vi "Teleop.vi"(10 "Match Info":T1={"Autonomous Elapsed Seconds"=0.0, "TeleOp Elapsed Seconds"=0.0, "Disabled Elapsed Seconds"=0.0, "Visited Autonomous"=FALSE, "Visited TeleOp"=FALSE, "Visited Disabled"=FALSE, "Autonomous Settings"={"Autonomous Style"=enum."Independent", "VI Refnum"=refnum}}, 11 "Call Context":T2) -> ()   [LabVIEW 2017]
doc: "This VI is called for each TeleOp packet received from the DS where the robot is not disabled. It is often used to read from the joysticks and update I/O or to update setpoints for timed control loops. It should complete and return within 20 milliseconds or it may miss DS packets."
uses:
  <vilib>/Rock Robotics/WPI/DriverStation/WPI_DriverStationDerivedRobotMode.ctl
  <vilib>/Rock Robotics/WPI/DriverStation/WPI_DriverStationMatch Info.ctl
  <vilib>/Rock Robotics/WPI/Solenoid/WPI_SolenoidValue.ctl
  Robot Global Data.vi
  <vilib>/Rock Robotics/Network Tables/NT Write Boolean Array.vi
  <vilib>/Rock Robotics/Network Tables/NT Write Numeric Array.vi
  <vilib>/Rock Robotics/WPI/Utilities/WPI_GetSetVariantRefNum.vi
  <vilib>/Rock Robotics/Network Tables/NT Read Boolean.vi
  <vilib>/Rock Robotics/Network Tables/NT Read String.vi
  <vilib>/Rock Robotics/WPI/Solenoid/WPI_SolenoidSetEnum.vi
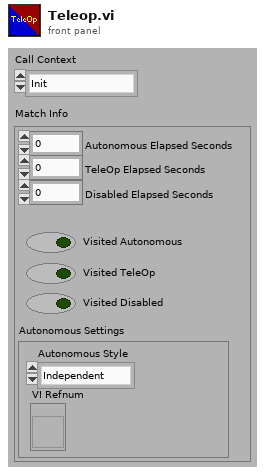
[diagram p1: front panel]
types:
  T1 = typedef "WPI_DriverStationMatch Info.ctl" = cluster{"Autonomous Elapsed Seconds":dbl, "TeleOp Elapsed Seconds":dbl, "Disabled Elapsed Seconds":dbl, "Visited Autonomous":bool, "Visited TeleOp":bool, "Visited Disabled":bool, "Autonomous Settings":cluster{"Autonomous Style":enum16{"Iterative", "Independent"}, "VI Refnum":refnum<vi>}}
  T2 = typedef "WPI_DriverStationDerivedRobotMode.ctl" = enum16{"Init", "Execute", "Stop"}
  T3 = enum16{"1 Xbox Controller", "2 Xbox Controllers"}
  T4 = typedef "TeleopCommands.ctl" = cluster{"Drive Axes":dbl[], "Shooter Forwards":bool, "Shooter Reverse":bool, "Intake Forwards":bool, "Intake Reverse":bool, "Lift Forwards":bool, "Lift Reverse":bool, "Agitator Forwards":bool, "Agitator Reverse":bool, "Left Gear Angle":bool, "Mid Gear Angle":bool, "Right Gear Angle":bool, "Shooter Distance":bool, "Vision Align":bool, "Place Gear":bool, "Command Stop":bool, "Reset Gyro":bool, "Jog Mode?":bool, "Lift Override":bool, "Lift Power":dbl}
  T5 = typedef "WPI_JoystickDevRef.ctl" = cluster{"Device":T6}
  T6 = typedef "WPI_JoystickDeviceEnum.ctl" = enum16{"USB 0", "USB 1", "USB 2", "USB 3", "USB 4", "USB 5"}
  T7 = cluster{"Yaw":dbl, "Roll":dbl, "Pitch":dbl, "Heading":dbl, "Fused Heading":dbl}
  T8 = typedef "WPI_MotorControlDeviceRef.ctl" = cluster{"DeviceStatus":errorcluster, "Type":T9, "PWM":cluster{"PWM Channel":T10, "DeadBand":T11}, "CAN":cluster{"Device Number":u8, "SetOutput VI Ref":variant, "GetOutput VI Ref":variant, "Enable VI Ref":variant, "Disable VI Ref":variant, "Data":variant}, "Invert":bool, "DIO PWM":cluster{"PWM \"Enable\" Channel":T10, "DIOChannel":T12, "PWM Rate":dbl}}
  T9 = typedef "WPI_MotorControlType.ctl" = enum16{"PWM", "CAN", "DIO PWM"}
  T10 = typedef "FPGA_DIOPWMChannel.ctl" = enum8{"PWM 0", "PWM 1", "PWM 2", "PWM 3", "PWM 4", "PWM 5", "PWM 6", "PWM 7", "PWM 8", "PWM 9", "PWM MXP 0", "PWM MXP 1", "PWM MXP 2", "PWM MXP 3", "PWM MXP 4", "PWM MXP 5", "PWM MXP 6", "PWM MXP 7", "PWM MXP 8", "PWM MXP 9", "Invalid"}
  T11 = typedef "WPI_PWMDeadband.ctl" = cluster{"Name":string, "maxPositivePwm":i32, "minPositivePwm":i32, "centerPwm":i32, "maxNegativePwm":i32, "minNegativePwm":i32, "angularRange":u16}
  T12 = typedef "FPGA_DIOChannel.ctl" = enum8{"DIO 0", "DIO 1", "DIO 2", "DIO 3", "DIO 4", "DIO 5", "DIO 6", "DIO 7", "DIO 8", "DIO 9", "DIO MXP 0", "DIO MXP 1", "DIO MXP 2", "DIO MXP 3", "DIO MXP 4", "DIO MXP 5", "DIO MXP 6", "DIO MXP 7", "DIO MXP 8", "DIO MXP 9", "DIO MXP 10", "DIO MXP 11", "DIO MXP 12", "DIO MXP 13", "DIO MXP 14", "DIO MXP 15", "SPI Port CS1", "SPI Port CS2", "SPI Port CS3", "SPI Port MISO", "SPI Port MOSI", "Invalid"}
  T13 = typedef "WPI_SolenoidDevRef.ctl" = cluster{"DevStatus":errorcluster, "Pneumatics Control Module":u8, "Forward Solenoid Channel":T14, "Reverse Solenoid Channel":T14}
  T14 = typedef "WPI_SolenoidChannel.ctl" = enum8{"Solenoid 0", "Solenoid 1", "Solenoid 2", "Solenoid 3", "Solenoid 4", "Solenoid 5", "Solenoid 6", "Solenoid 7", "Invalid"}
  T15 = typedef "WPI_SolenoidValue.ctl" = enum16{"Off", "On", "Forward", "Reverse"}
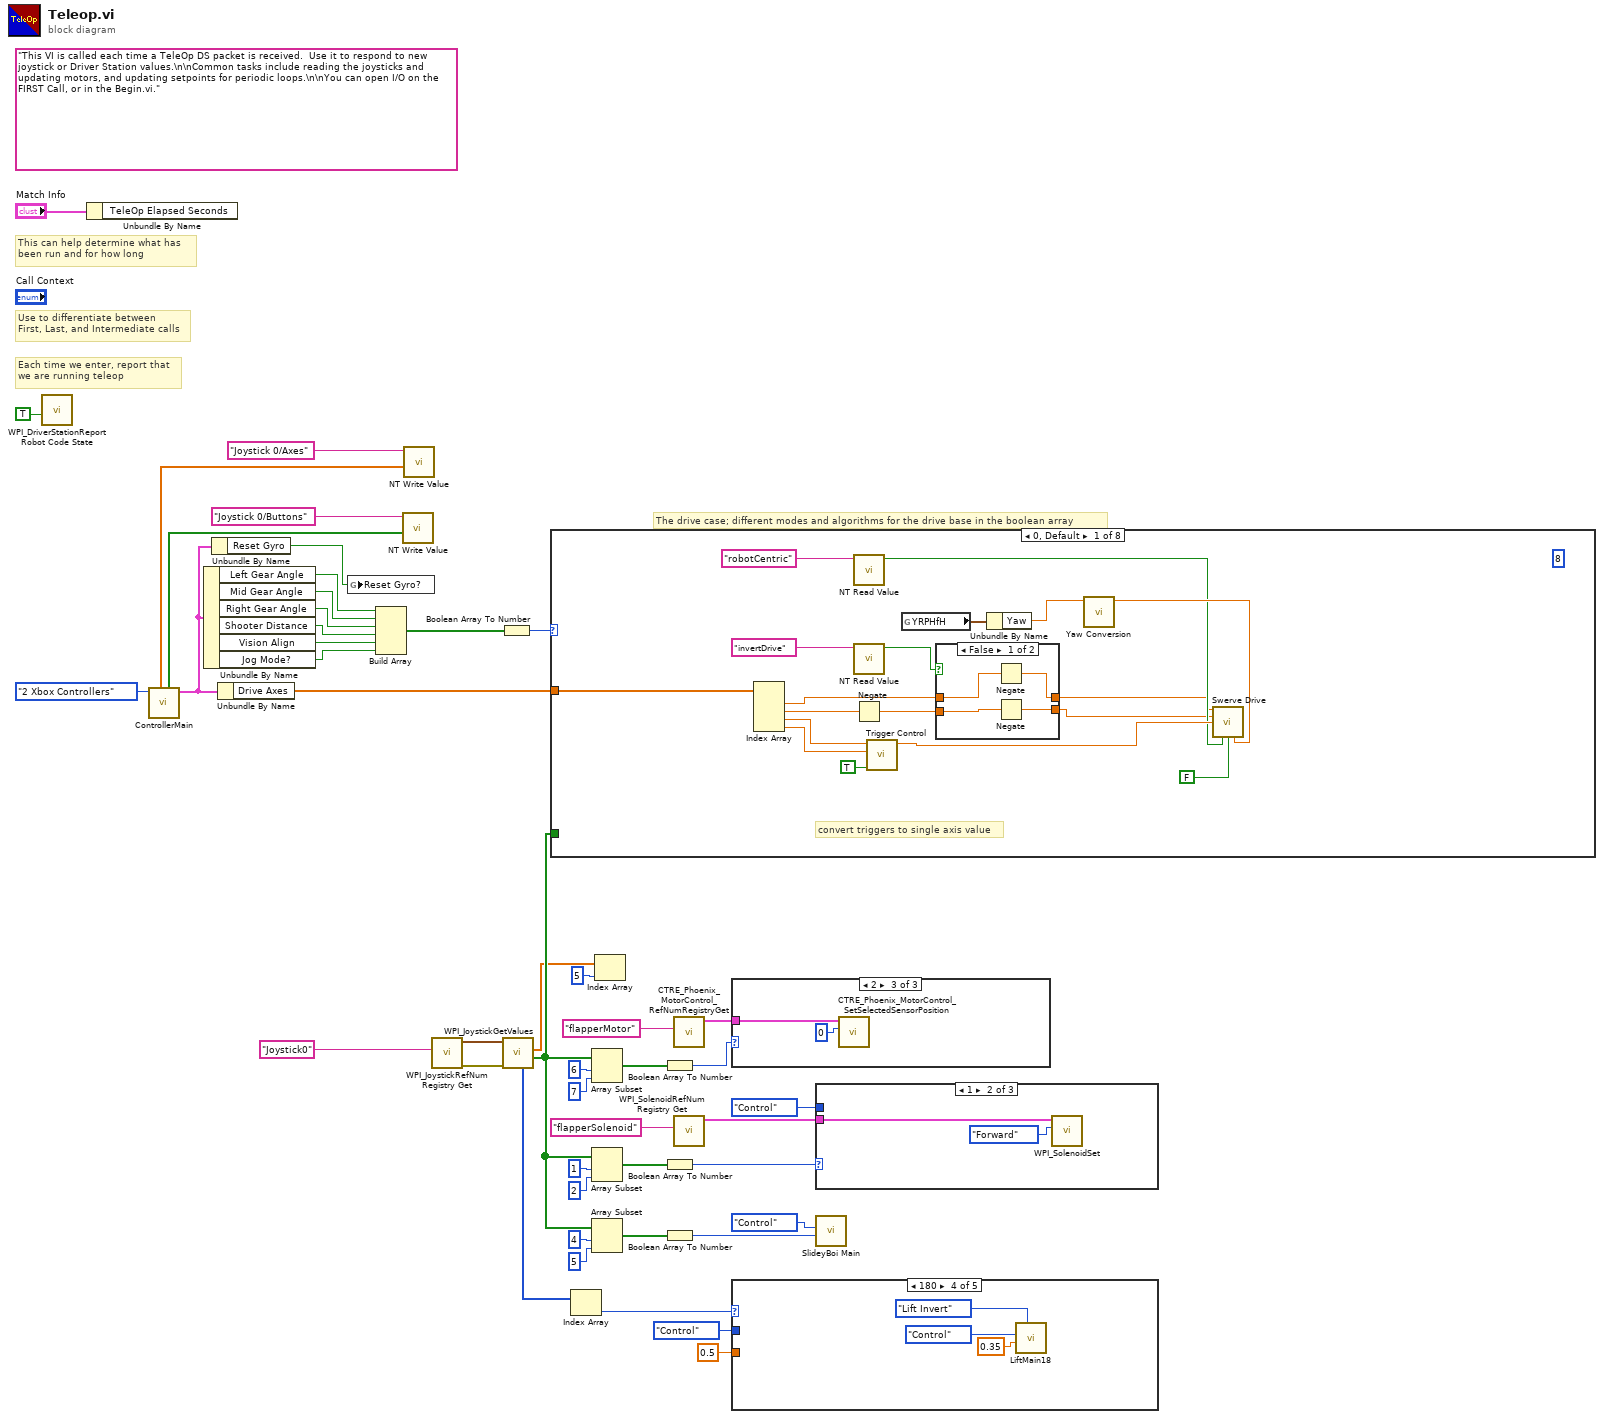
[diagram p0: block diagram]
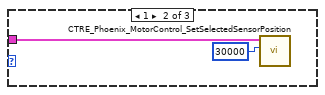
[diagram p3: hidden frame]
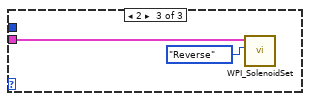
[diagram p5: hidden frame]
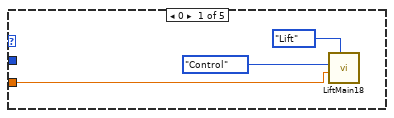
[diagram p6: hidden frame]
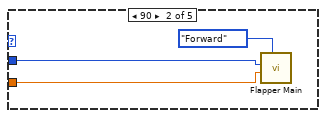
[diagram p7: hidden frame]
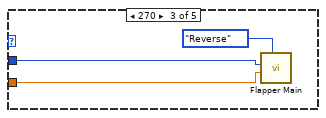
[diagram p8: hidden frame]
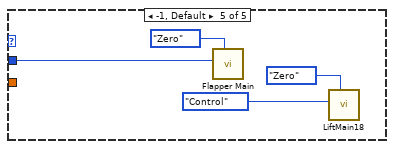
[diagram p9: hidden frame]
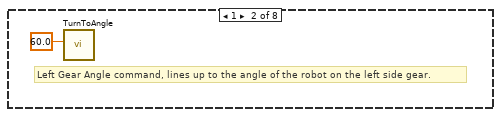
[diagram p11: hidden frame]
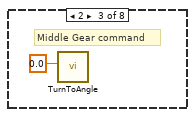
[diagram p12: hidden frame]
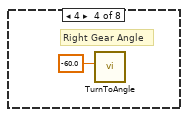
[diagram p13: hidden frame]
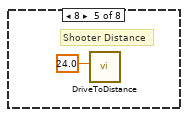
[diagram p14: hidden frame]
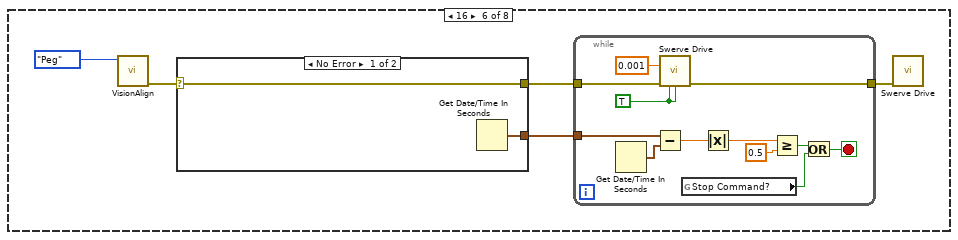
[diagram p15: hidden frame]
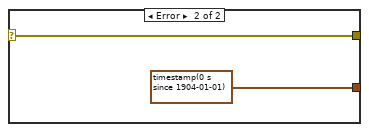
[diagram p16: hidden frame]
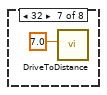
[diagram p17: hidden frame]
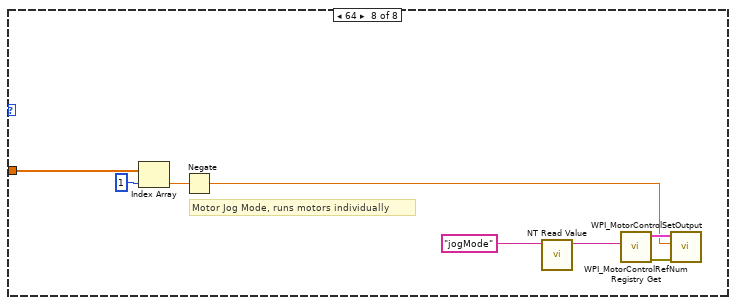
[diagram p18: hidden frame]
diagram:
  (unwired) "This VI is called each time a TeleOp DS packet is received.  Use it to respond to new joystick or Driver Station values.\n\nCommon tasks include reading the joysticks and updating motors, and updating setpoints for periodic loops.\n\nYou can open I/O on the FIRST Call, or in the Begin.vi."
  # "The drive case; different modes and algorithms for the drive base in the boolean array"
  # "Each time we enter, report that\nwe are running teleop"
  # "Use to differentiate between\nFirst, Last, and Intermediate calls"
  # "This can help determine what has\nbeen run and for how long"
  n1 = call <vilib>:"WPI_DriverStationReport Robot Code State.vi"("TeleOp"=TRUE ("Autonomous")) -> ()  [unwired: 10 in, 1 out]
  n2 = Unbundle By Name("Match Info") -> ()  [unwired: 1 out]
  n3 = call "ControllerMain.vi"("Control Mode"=T3."2 Xbox Controllers") -> ("Robot Inputs"=w39:T4, "Stick0 Buttons"=w42:bool[], "Stick0 Axes"=w43:dbl[])  [unwired: 5 in, 3 out]
  n4 = Unbundle By Name(w39) -> ("Left Gear Angle"=w37:bool, "Mid Gear Angle"=w36:bool, "Right Gear Angle"=w35:bool, "Shooter Distance"=w34:bool, "Vision Align"=w33:bool, "Jog Mode?"=w32:bool)
  n5 = Unbundle By Name(w39) -> ("Reset Gyro"=w38:bool)
  n6 = Unbundle By Name(w39) -> ("Drive Axes"=w29:dbl[])
  n7 = global write "Robot Global Data.vi" "Reset Gyro?"(w38) -> ()
  n8 = Build Array(w37, w36, w35, w34, w33, w32) -> (w31:bool[])
  n9 = call-poly <vilib>:"NT Write Value.vi"("Boolean Array"=w42, "Name"="Joystick 0/Buttons") -> ()  [unwired: 9 in, 1 out]
  n10 = call-poly <vilib>:"NT Write Value.vi"("Numeric Array"=w43, "Name"="Joystick 0/Axes") -> ()  [unwired: 9 in, 1 out]
  n11 = call <vilib>:"WPI_JoystickRefNum Registry Get.vi"("refnum name"="Joystick0") -> ("error out"=w27:errorcluster, "JoystickDevRef"=w26:T5)  [unwired: 9 in]
  n12 = Boolean Array To Number(Boolean array=w31) -> (number=w30:u32)
  n13 = call <vilib>:"WPI_JoystickGetValues.vi"("error in (no error)"=w27, "JoystickDevRef"=w26) -> ("Buttons"=w4:bool[], "Axes"=w3:dbl[], "POVs"=w25:i16[])  [unwired: 5 in, 2 out]
  n14 = case shown="0, Default" w30 {
    tunnel: w29 -> [w62 _ _ _ _ _ _ w104]
    tunnel: w4 -> [_ _ _ _ _ _ _ _]
    frame 0, Default {
      (unwired) 8 ("index")
      # "convert triggers to single axis value"
      n15 = Index Array(array=w62) -> (element #1=w54:dbl, element #2=w52:dbl, element #3=w61:dbl, element #4=w60:dbl)  [unwired: 4 in]
      n16 = call-poly <vilib>:"NT Read Value.vi"("Name"="robotCentric") -> ("Boolean"=w49:bool)  [unwired: 9 in, 1 out]
      n17 = call-poly <vilib>:"NT Read Value.vi"("Name"="invertDrive") -> ("Boolean"=w63:bool)  [unwired: 9 in, 1 out]
      n18 = Negate(x=w52) -> (-x=w53:dbl)
      n19 = call "Trigger Control.vi"("Invert?"=TRUE, "Axis 2 In"=w60, "Axis 1 In"=w61) -> ("Axis Out"=w56:dbl)  [unwired: 8 in]
      n20 = global read "Robot Global Data.vi" "YRPHfH"() -> (w58:T7)
      n21 = case shown="False" w63 {
        tunnel: w53 -> [w68 w70]
        tunnel: w54 -> [w67 w69]
        tunnel: [w66 w70] -> w48
        tunnel: [w65 w69] -> w47
        frame False {
          n22 = Negate(x=w67) -> (-x=w65:dbl)
          n23 = Negate(x=w68) -> (-x=w66:dbl)
        }
        frame True {
        }
      }
      n24 = Unbundle By Name(w58) -> ("Yaw"=w51:dbl)
      n25 = call "Yaw Conversion.vi"("Input"=w51) -> ("Output"=w50:dbl)  [unwired: 10 in]
      n26 = call "Swerve Drive.vi"("X"=w47, "Y"=w48, "Z"=w56, "Robot Centric?"=w49, "Autonomous?"=FALSE ("Robot Centric?"), "Yaw"=w50) -> ()  [unwired: 5 in, 5 out]
    }
    frame 1 {
      # "Left Gear Angle command, lines up to the angle of the robot on the left side gear."
      n27 = call "TurnToAngle.vi"("Target Angle"=60.0) -> ()  [unwired: 10 in, 1 out]
    }
    frame 2 {
      # "Middle Gear command"
      n28 = call "TurnToAngle.vi"("Target Angle"=0.0) -> ()  [unwired: 10 in, 1 out]
    }
    frame 4 {
      # "Right Gear Angle"
      n29 = call "TurnToAngle.vi"("Target Angle"=-60.0) -> ()  [unwired: 10 in, 1 out]
    }
    frame 8 {
      # "Shooter Distance"
      n30 = call "DriveToDistance.vi"("Setpoint"=24.0) -> ()  [unwired: 10 in, 1 out]
    }
    frame 16 {
      n31 = call "VisionAlign.vi"("Control Mode"=enum16{"Boiler", "Peg"}."Peg") -> ("Error Out"=w78:errorcluster)  [unwired: 10 in]
      n32 = case shown="No Error" w78 {
        selector: w78 -> [w93 w94]
        tunnel: [w93 w94] -> w76
        tunnel: [w92 timestamp(0 s since 1904-01-01)] -> w77
        frame No Error {
          n33 = Get Date/Time In Seconds() -> (seconds since 1Jan1904=w92:timestamp)
        }
        frame Error {
        }
      }
      n34 = while {
        tunnel: w77 -> [w91]
        tunnel: w76 -> [w85]
        tunnel: [w80] -> w75
        stop <- w81 stop-if-true
        w86 = TRUE ("Robot Centric?")
        n35 = Get Date/Time In Seconds() -> (seconds since 1Jan1904=w90:timestamp)
        n36 = Subtract(x=w91, y=w90) -> (x-y=w89:dbl)
        n37 = call "Swerve Drive.vi"("Y"=0.001, "Error In"=w85, "Robot Centric?"=w86, "Autonomous?"=w86) -> ("Error Out"=w80:errorcluster)  [unwired: 7 in, 4 out]
        n38 = global read "Robot Global Data.vi" "Stop Command?"() -> (w82:bool)
        n39 = Absolute Value(x=w89) -> (abs(x)=w88:dbl)
        n40 = Greater Or Equal?(x=w88, y=0.5) -> (x >= y?=w83:bool)
        n41 = Or(x=w83, y=w82) -> (x .or. y?=w81:bool)
      }
      n42 = call "Swerve Drive.vi"("Error In"=w75) -> ()  [unwired: 10 in, 5 out]
    }
    frame 32 {
      n43 = call "DriveToDistance.vi"("Setpoint"=7.0) -> ()  [unwired: 10 in, 1 out]
    }
    frame 64 {
      # "Motor Jog Mode, runs motors individually"
      n44 = Index Array(array=w104, index=1) -> (element=w102:dbl)
      n45 = Negate(x=w102) -> (-x=w98:dbl)
      n46 = call-poly <vilib>:"NT Read Value.vi"("Name"="jogMode") -> ("String"=w97:string)  [unwired: 9 in, 1 out]
      n47 = call <vilib>:"WPI_MotorControlRefNum Registry Get.vi"("refnum name"=w97) -> ("error out"=w99:errorcluster, "MotorControlDevRef"=w100:T8)  [unwired: 9 in]
      n48 = call <vilib>:"WPI_MotorControlSetOutput.vi"("error in (no error)"=w99, "Output"=w98, "MotorControlDevRef"=w100) -> ()  [unwired: 6 in, 3 out]
    }
  }
  n49 = Index Array(array=w25) -> (element=w24:i16)  [unwired: 1 in]
  n50 = Array Subset(array=w4, index=6, length=7) -> (w8:bool[])
  n51 = Array Subset(array=w4, index=1, length=2) -> (w21:bool[])
  n52 = Array Subset(array=w4, index=4, length=5) -> (w20:bool[])
  n53 = Index Array(array=w3, index=5) -> ()  [unwired: 1 out]
  n54 = Boolean Array To Number(Boolean array=w8) -> (number=w7:u32)
  n55 = Boolean Array To Number(Boolean array=w21) -> (number=w14:u32)
  n56 = Boolean Array To Number(Boolean array=w20) -> (number=w16:u32)
  n57 = call <vilib>:"CTRE_Phoenix_MotorControl_RefNumRegistryGet.vi"("refnum name"="flapperMotor") -> ("PhoenixMotorControlDevRef"=w5:T8)  [unwired: 9 in, 1 out]
  n58 = call <vilib>:"WPI_SolenoidRefNum Registry Get.vi"("refnum name"="flapperSolenoid") -> ("SolenoidDevRef"=w11:T13)  [unwired: 9 in, 1 out]
  n59 = case shown="2" w7 {
    tunnel: w5 -> [_ w106 w108]
    frame 0, Default {
    }
    frame 1 {
      n60 = call <vilib>:"CTRE_Phoenix_MotorControl_SetSelectedSensorPosition.vi"("New Sensor Position"=30000, "PhoenixMotorControlDevRef"=w106) -> ()  [unwired: 8 in, 2 out]
    }
    frame 2 {
      n61 = call <vilib>:"CTRE_Phoenix_MotorControl_SetSelectedSensorPosition.vi"("New Sensor Position"=0, "PhoenixMotorControlDevRef"=w108) -> ()  [unwired: 8 in, 2 out]
    }
  }
  n62 = case shown="180" w24 {
    tunnel: enum16{"Open", "Control"}."Control" ("Control Mode") -> [_ w114 w117 _ w122]
    tunnel: 0.5 ("Power") -> [w109 w112 w115 _ _]
    frame 0 {
      n63 = call "LiftMain18.vi"("Operation Mode"=enum16{"Lift", "Lift Invert", "Zero"}."Lift", "Power"=w109, "Control Mode"=enum16{"Open", "Control"}."Control") -> ()  [unwired: 9 in]
    }
    frame 90 {
      n64 = call "Flapper Main.vi"("Control Options"=enum16{"Zero", "Forward", "Reverse"}."Forward", "Power"=w112, "Control Mode"=w114) -> ()  [unwired: 9 in]
    }
    frame 270 {
      n65 = call "Flapper Main.vi"("Control Options"=enum16{"Zero", "Forward", "Reverse"}."Reverse", "Power"=w115, "Control Mode"=w117) -> ()  [unwired: 9 in]
    }
    frame 180 {
      n66 = call "LiftMain18.vi"("Operation Mode"=enum16{"Lift", "Lift Invert", "Zero"}."Lift Invert", "Power"=0.35, "Control Mode"=enum16{"Open", "Control"}."Control") -> ()  [unwired: 9 in]
    }
    frame -1, Default {
      n67 = call "Flapper Main.vi"("Control Options"=enum16{"Zero", "Forward", "Reverse"}."Zero", "Control Mode"=w122) -> ()  [unwired: 10 in]
      n68 = call "LiftMain18.vi"("Operation Mode"=enum16{"Lift", "Lift Invert", "Zero"}."Zero", "Control Mode"=enum16{"Open", "Control"}."Control") -> ()  [unwired: 10 in]
    }
  }
  n69 = case shown="1" w14 {
    tunnel: enum16{"Open", "Control"}."Control" ("Control Mode") -> [_ _ _]
    tunnel: w11 -> [_ w126 w127]
    frame 0, Default {
    }
    frame 1 {
      n70 = call-poly <vilib>:"WPI_SolenoidSet.vi"("Value"=WPI_SolenoidValue."Forward", "SolenoidDevRef"=w126) -> ()  [unwired: 8 in, 2 out]
    }
    frame 2 {
      n71 = call-poly <vilib>:"WPI_SolenoidSet.vi"("Value"=WPI_SolenoidValue."Reverse", "SolenoidDevRef"=w127) -> ()  [unwired: 8 in, 2 out]
    }
  }
  n72 = call "SlideyBoi Main.vi"("Control Option"=w16, "Control Mode"=enum16{"Open", "Control"}."Control") -> ()  [unwired: 10 in]
